vi "Get Register.vi"(11 "Actor in":refnum<class "Actor.lvclass">) -> (2 "Register":refnum<event-registration>)   [LabVIEW 2021, in "jettl.lvlib" / "Actor.lvlib" / "Actor.lvclass"]
uses:
  Actor.lvclass
  Msg/Msg.lvclass
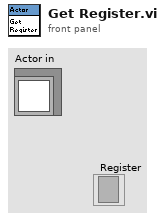
[diagram p1: front panel]
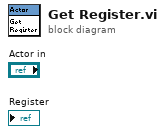
[diagram p0: block diagram]
diagram:
